vi "Execute Dig.vi"(6 "Mouse Position":T1, 8 "User VI Ref":refnum<vi>, 9 "Menu Item Tag Suffix":string, 10 "Remaining Items":refnum<vi>[](array[refnum]), 11 "Affected Items":T2) -> (0 "Fail transaction?":bool)   [LabVIEW 2017, in "Shortcut Menu.lvlib"]
doc: "This VI is part of a plug-in for modifying the LabVIEW shortcut menus. This is the execute VI which is called when the shortcut menu is chosen by the user. It performs the action of the selected menu item."
uses:
  Shortcut Menu.lvlib
  Dig.ctl
  <vilib>/Utility/miscctls.llb/LVPositionTypeDef.ctl
  Eulogy/Eulogy.lvlib
panel:
  # "All controls on this panel except \"Affected Items\" have been locked to prevent accidental edits. Changing the control names or types, other than the elements of the \"Affected Items\" cluster will make the VI unusable as a menu plugin.\n\nSee Context Help for each control for details about its use."
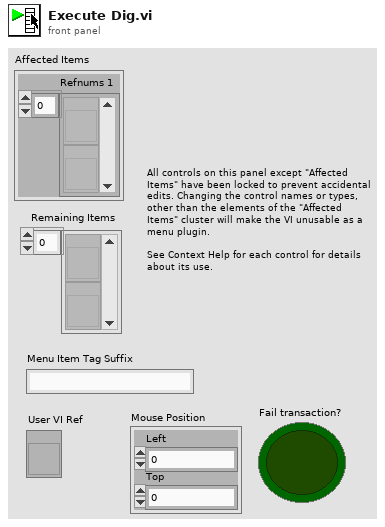
[diagram p1: front panel]
types:
  T1 = typedef "LVPositionTypeDef.ctl" = cluster{"Left":i32, "Top":i32}
  T2 = typedef "Shortcut Menu.lvlib/Dig.ctl" = cluster{"Refnums 1":refnum<vi>[]}
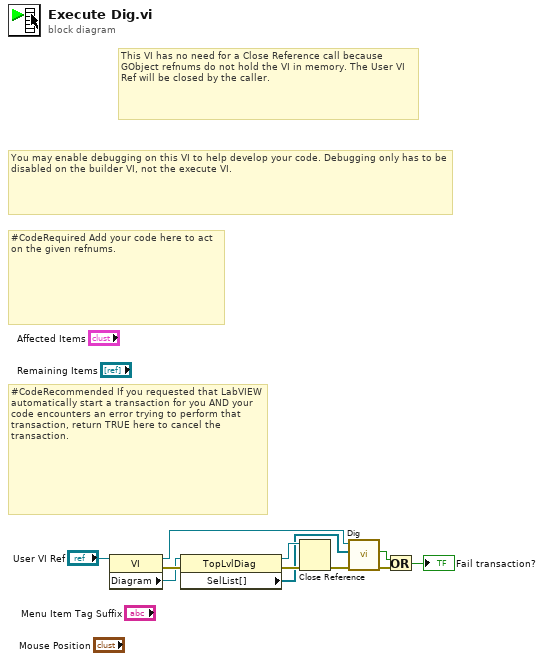
[diagram p0: block diagram]
diagram:
  # "You may enable debugging on this VI to help develop your code. Debugging only has to be disabled on the builder VI, not the execute VI."
  # "#CodeRecommended If you requested that LabVIEW automatically start a transaction for you AND your code encounters an error trying to perform that transaction, return TRUE here to cancel the transaction."
  # "#CodeRequired Add your code here to act on the given refnums."
  # "This VI has no need for a Close Reference call because GObject refnums do not hold the VI in memory. The User VI Ref will be closed by the caller."
  n1 = property class="VI"(reference="User VI Ref") -> (reference out=w4:refnum<vi>, error out=w8:errorcluster, "Diagram"=w7:refnum<vi>)  [unwired: 1 in]
  n2 = property class="TopLvlDiag"(reference=w7, error in=w8) -> (reference out=w5:refnum<vi>, error out=w6:errorcluster, "SelList[]"=w3:refnum<vi>[])
  n3 = Close Reference(reference=w5, error in (no error)=w6) -> (error out=w2:errorcluster)
  n4 = call "Dig.vi"("Error In"=w2, "Selection List[]"=w3, "VI In"=w4) -> ("Error Out"=w11:errorcluster, "Change Made?"=w1:bool)  [unwired: 6 in, 1 out]
  n5 = Or(x=w1, y=w11) -> (x .or. y?=→"Fail transaction?":bool)
